vi "Boiler.vi"() -> ()   [LabVIEW 2013]
doc: "This VI is a simulaton of boiler startup controller which allow the user to Start up and Shutdown a boiler.\n\nThe controls on the front panal is to- \n-Start up \n-Simulate the cindition in system and\n-Shut down .\nThe indicators on the front panal is to-\n-Display the status and current step in the startup\n-Display the Shut down process\n-Shoe the elapsed time\n\nThis controller also log event the event as thry occur.\n\nSequence of operation:\n-Start(Application Run): This will start the application and initialize all the controls and indicator.\n-Reset Lockout: This will ready the boiler (It will happen only when Run interlock is in off position).\n-Pre-Purge: On pressing Start sequence this will run for 10 sec.\n-Pilot: On pressing pilot and it will start when Flame senseor value is more than 30%.\n-Shutdown: On pressing it the boiler will go in shut down and it can be done in four ways-\n>shutdoen is clicked\n>Fuel controller value is less than 10% or greater than 75%\n>Run itnterlock switch open.\n>Forced draft switch Off."
uses:
  Controls/Boiler Controls.ctl
  Controls/Boiler Simulation Controls.ctl
  Controls/Boiler Status Indicators.ctl
  Controls/Boiler Application Controls.ctl
  Controls/Boiler States.ctl
panel:
  in  "Stop":T1
  out "Boiler Status Indicators":T2 {"Time Count" format="%.2g"}
  in  "Boiler Simulation Controls":T3 {"Flame Sensor Value (%)" min=0.0 max=100.0 scale=0.0..100.0}
  in  "Boiler Controls":T4 {"Fuel Valve Position" min=0.0 max=100.0 scale=0.0..100.0 scale format="%.2f"}
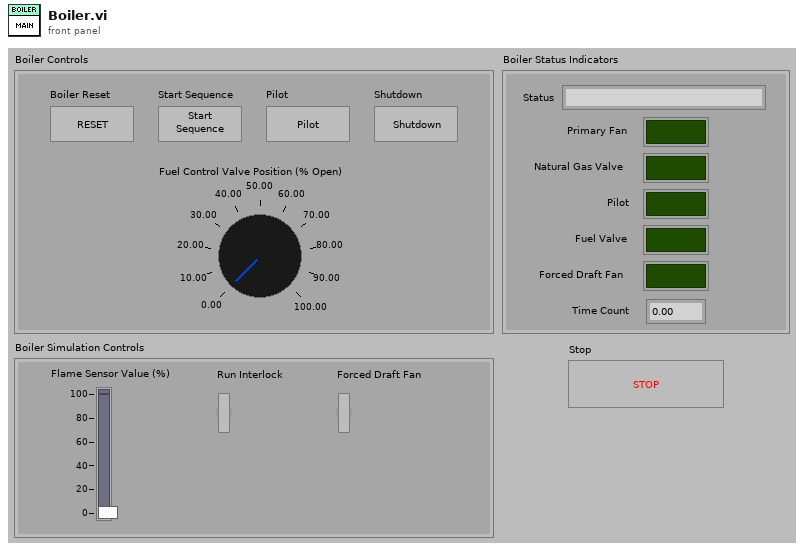
[diagram p1: front panel]
types:
  T1 = typedef "Boiler Application Controls.ctl" = bool
  T2 = typedef "Boiler Status Indicators.ctl" = cluster{"Status":string, "Primary Fan":bool, "Natural Gas Valve":bool, "Pilot":bool, "Fuel Valve":bool, "Forced Draft Fan":bool, "Time Count":dbl}
  T3 = typedef "Boiler Simulation Controls.ctl" = cluster{"Flame Sensor Value (%)":dbl, "Run Interlock":bool, "Forced Draft Fan":bool}
  T4 = typedef "Boiler Controls.ctl" = cluster{"Boiler Reset":bool, "Start Sequence":bool, "Pilot":bool, "Shutdown":bool, "Fuel Valve Position":dbl}
  T5 = typedef "Boiler States.ctl" = enum16{"Initialize", "Reset Lockout", "Pre-Purge", "Pre-Purge(Cont.)", "Ignition", "Prove the pilot", "Start and Run", "Run(Cont.) ", "Shutdown and purge", "Stop"}
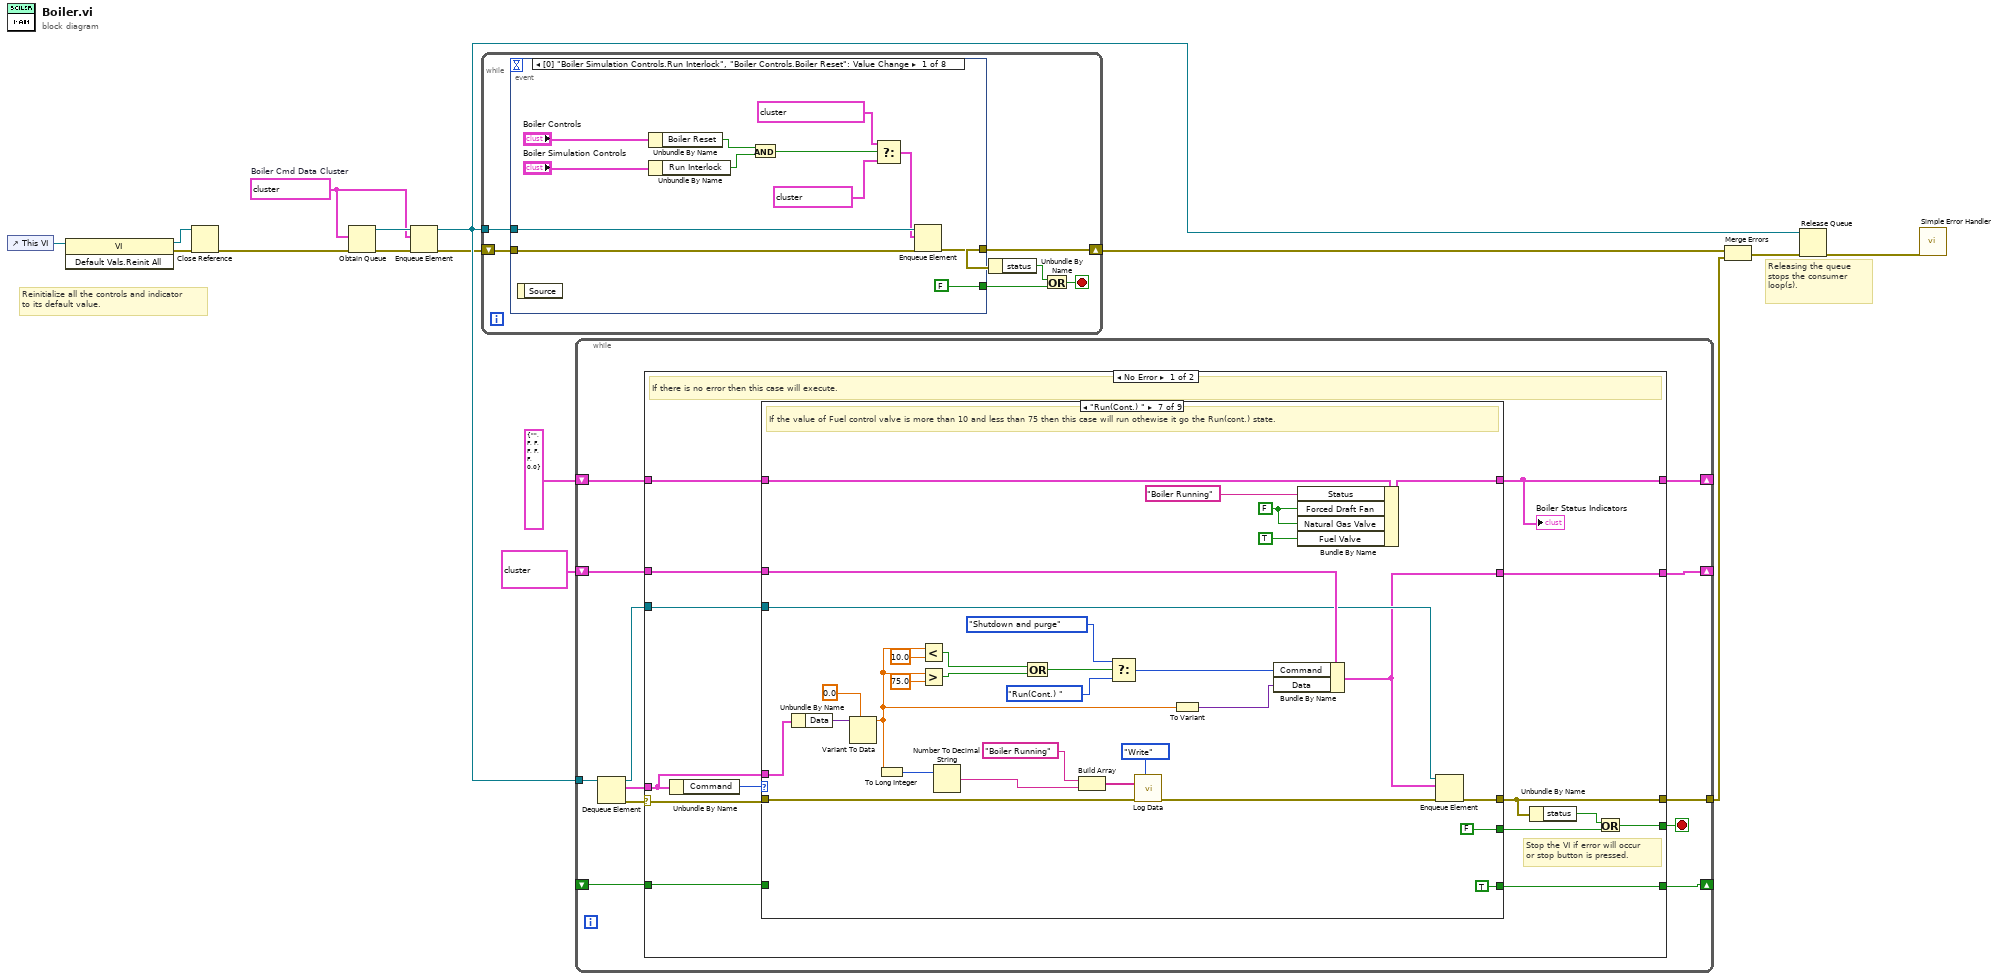
[diagram p0: block diagram]
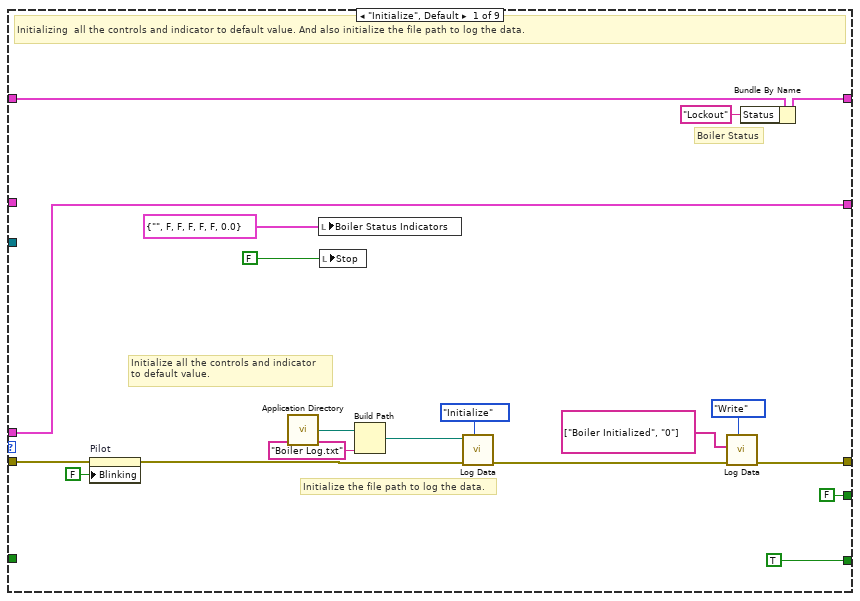
[diagram p2: hidden frame]
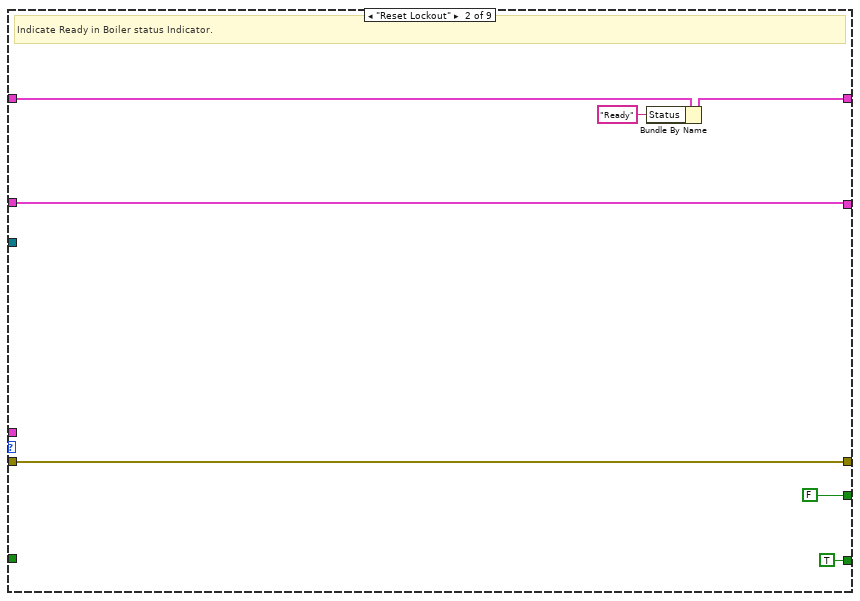
[diagram p3: hidden frame]
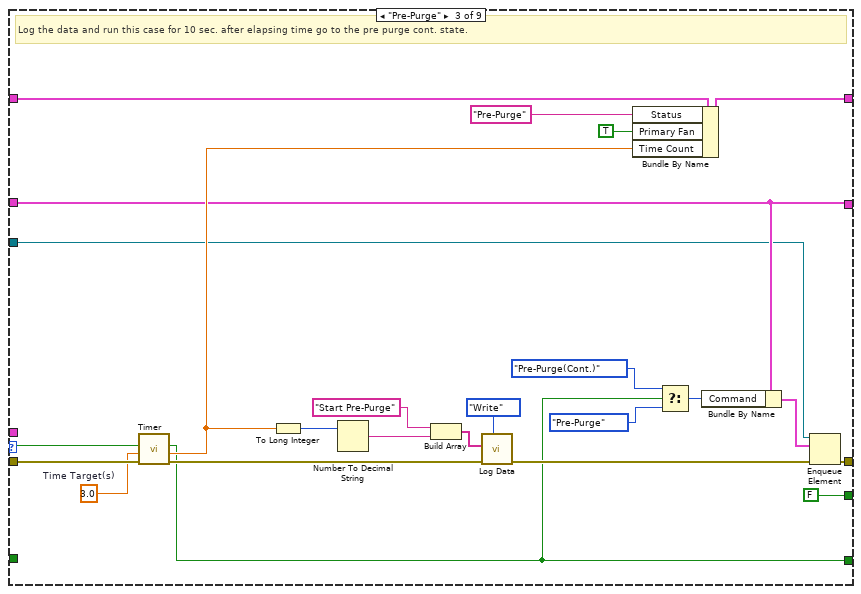
[diagram p4: hidden frame]
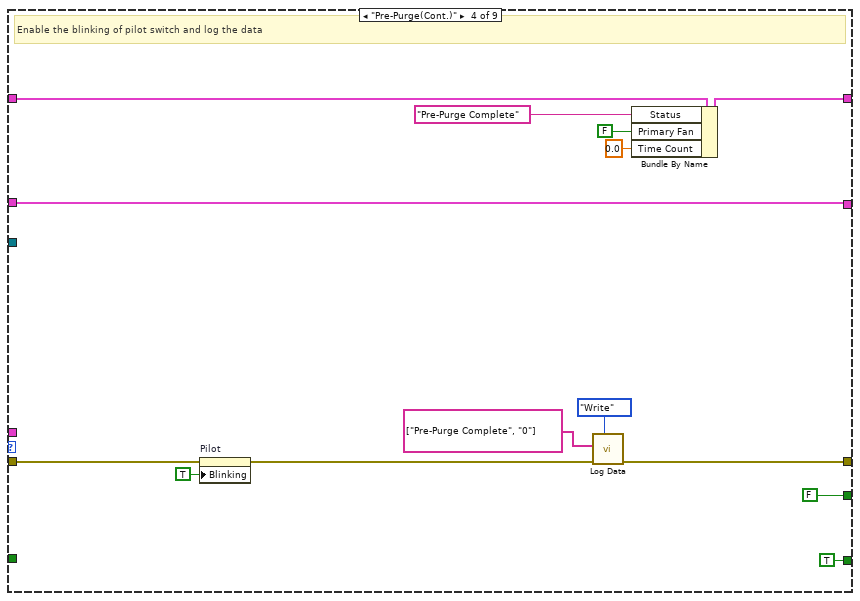
[diagram p5: hidden frame]
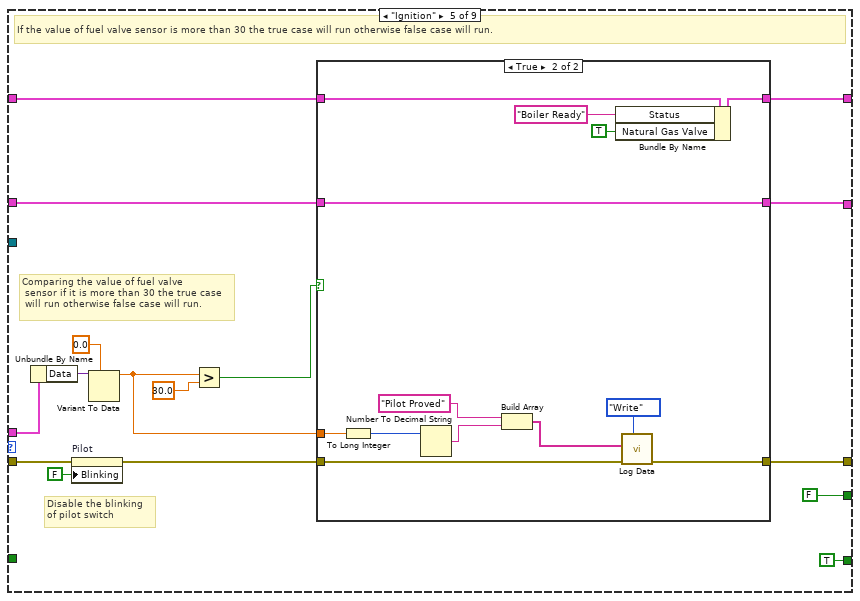
[diagram p6: hidden frame]
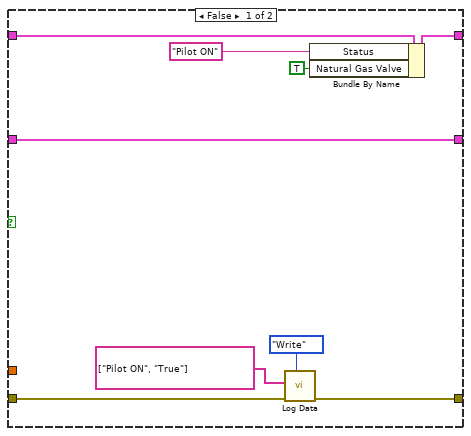
[diagram p7: hidden frame]
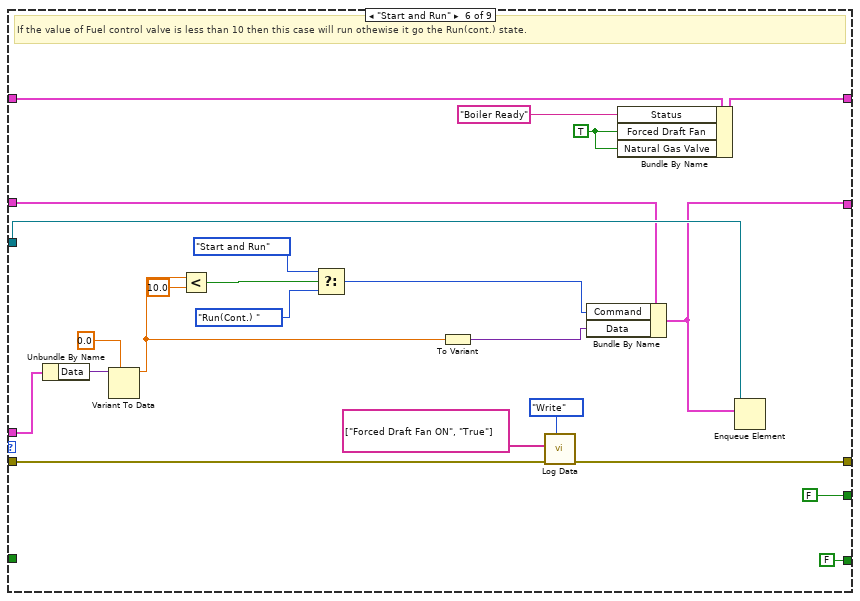
[diagram p8: hidden frame]
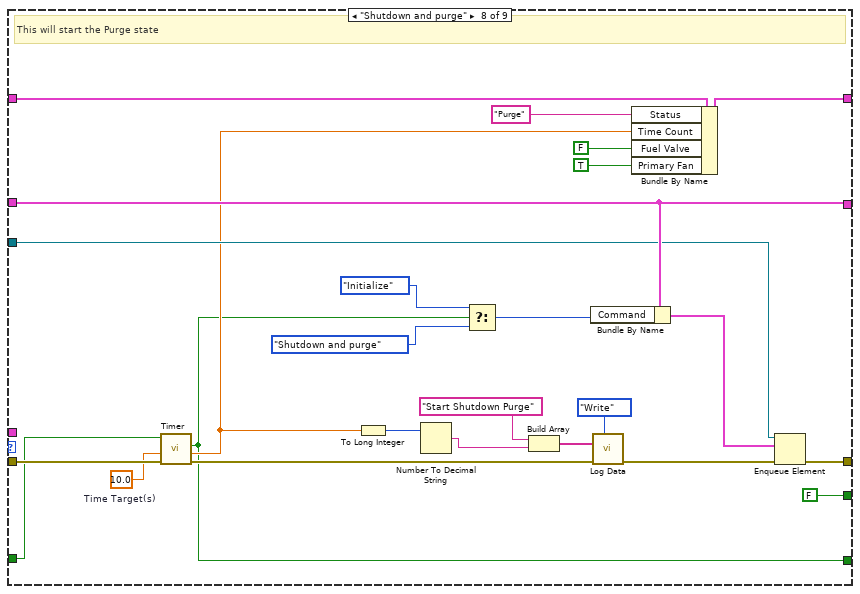
[diagram p9: hidden frame]
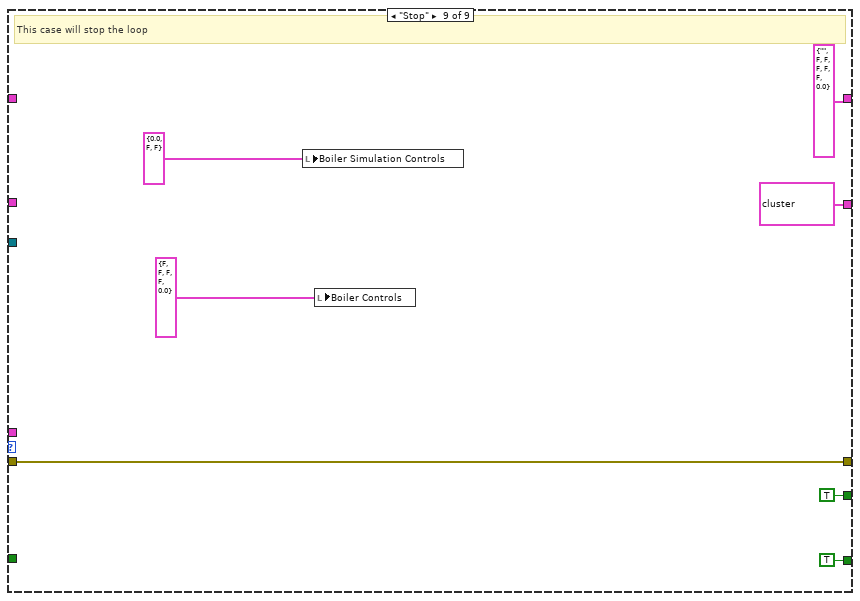
[diagram p10: hidden frame]
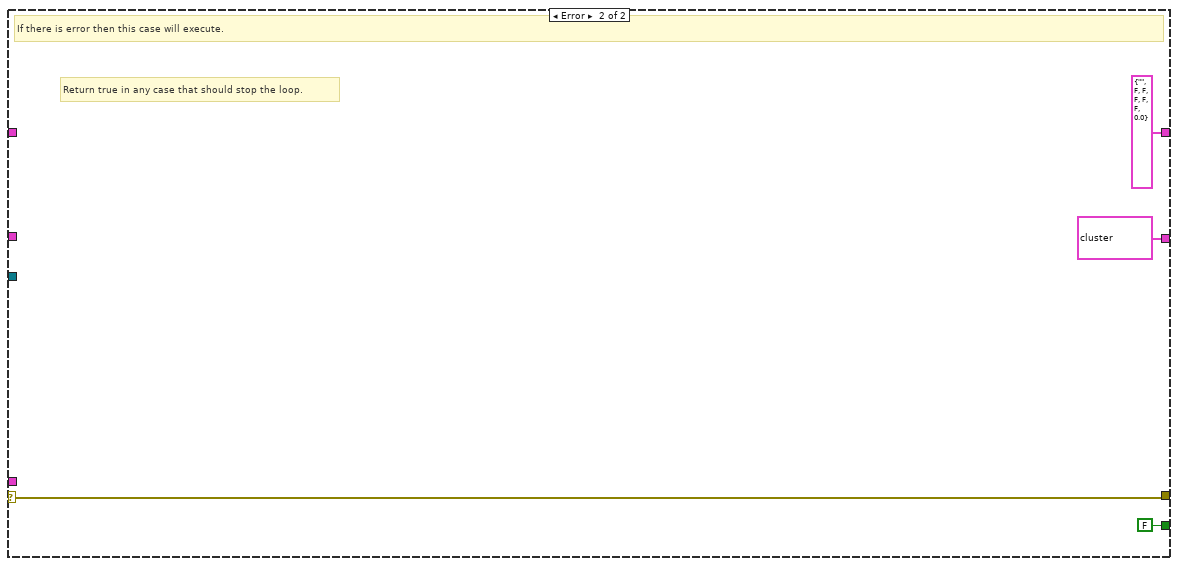
[diagram p11: hidden frame]
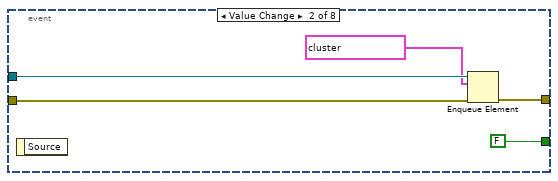
[diagram p12: hidden frame]
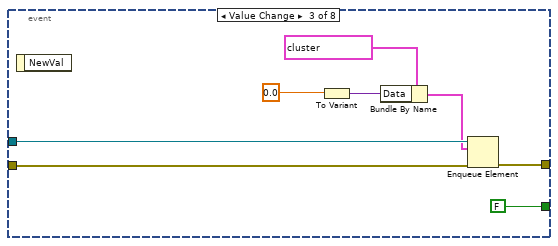
[diagram p13: hidden frame]
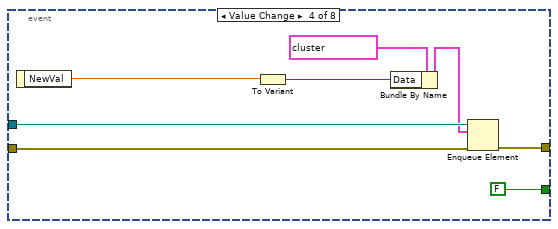
[diagram p14: hidden frame]
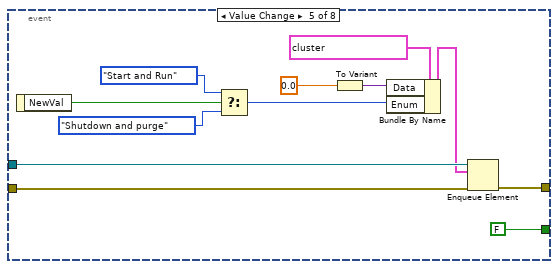
[diagram p15: hidden frame]
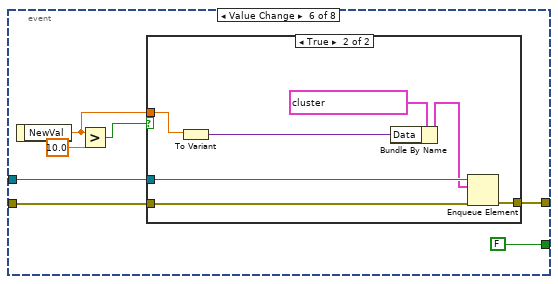
[diagram p16: hidden frame]
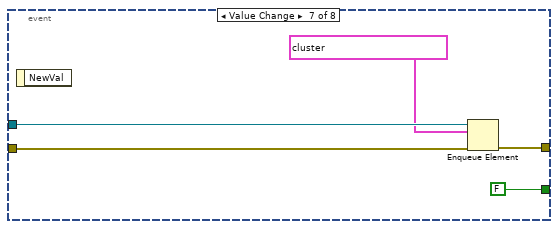
[diagram p18: hidden frame]
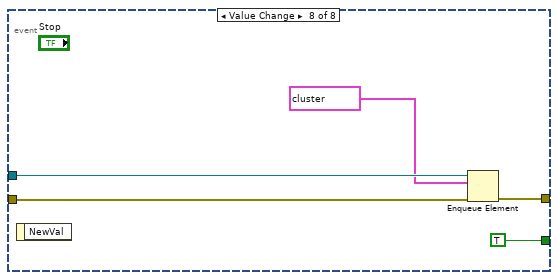
[diagram p19: hidden frame]
diagram:
  w7 = cluster{"Data":variant, "Command":T5} {"Data"=variant, "Command"=enum."Initialize"}  # Boiler Cmd Data Cluster
  # "Reinitialize all the controls and indicator\nto its default value."
  # "Releasing the queue stops the consumer loop(s)."
  n1 = control-ref of="This VI"() -> (w11:refnum<vi>)
  n2 = invoke class="VI" method="Default Vals.Reinit All"(reference=w11) -> (reference out=w9:refnum<vi>, error out=w10:errorcluster)  [unwired: 2 in, 1 out]
  n3 = Close Reference(reference=w9, error in (no error)=w10) -> (error out=w8:errorcluster)
  n4 = Obtain Queue(element data type=w7, error in (no error)=w8) -> (queue out=w15:refnum<queue>, error out=w13:errorcluster)  [unwired: 3 in, 1 out]
  n5 = Enqueue Element(queue=w15, element=w7, error in (no error)=w13) -> (queue out=w14:refnum<queue>, error out=w12:errorcluster)  [unwired: 1 in, 1 out]
  n6 = while {
    shift-right: [w18] -> w6
    shift-left: w12 -> [w20]
    tunnel: w14 -> [w21]
    stop <- w19 stop-if-true
    n7 = event shown="[0] \"Boiler Simulation Controls.Run Interlock\", \"Boiler Controls.Boiler Reset\": Value Change" {
      selector: _ -> [_ _ _ _ _ _ _ _]
      dyn-events: _ -> [_ _ _ _ _ _ _ _]
      timeout: _ -> [_ _ _ _ _ _ _ _]
      tunnel: w21 -> [w31 w36 w44 w52 w64 w71 w84 w89]
      tunnel: w20 -> [w33 w38 w46 w54 w66 w73 w86 w91]
      tunnel: [w32 w37 w45 w53 w65 w72 w85 w90] -> w18
      tunnel: [FALSE FALSE FALSE FALSE FALSE FALSE FALSE TRUE] -> w16
      event Value Change {
        n8 = event-data() -> ()  [unwired: 1 in, 1 out]
        n9 = Unbundle By Name("Boiler Controls") -> ("Boiler Reset"=w28:bool)
        n10 = Unbundle By Name("Boiler Simulation Controls") -> ("Run Interlock"=w29:bool)
        n11 = And(x=w28, y=w29) -> (x .and. y?=w27:bool)
        n12 = Select(t=cluster{"Data":variant, "Enum":T5} {"Data"=variant, "Enum"=enum."Reset Lockout"} ("Boiler Cmd Data Cluster"), s=w27, f=cluster{"Data":variant, "Enum":T5} {"Data"=variant, "Enum"=enum."Initialize"} ("Boiler Cmd Data Cluster")) -> (s? t:f=w24:cluster{"Data":variant, "Enum":T5})
        n13 = Enqueue Element(queue=w31, element=w24, error in (no error)=w33) -> (error out=w32:errorcluster)  [unwired: 1 in, 2 out]
      }
      event Value Change {
        n14 = event-data() -> ()  [unwired: 1 in, 1 out]
        n15 = Enqueue Element(queue=w36, element=cluster{"Data":variant, "Enum":T5} {"Data"=variant, "Enum"=enum."Pre-Purge"} ("Boiler Cmd Data Cluster"), error in (no error)=w38) -> (error out=w37:errorcluster)  [unwired: 1 in, 2 out]
      }
      event Value Change {
        n16 = event-data() -> ()  [unwired: 1 in, 1 out]
        n17 = To Variant(anything=0.0) -> (Variant=w39:variant)
        n18 = Bundle By Name(cluster=cluster{"Data":variant, "Enum":T5} {"Data"=variant, "Enum"=enum."Ignition"} ("Boiler Cmd Data Cluster"), "Data"=w39) -> (w41:cluster{"Data":variant, "Enum":T5})
        n19 = Enqueue Element(queue=w44, element=w41, error in (no error)=w46) -> (error out=w45:errorcluster)  [unwired: 1 in, 2 out]
      }
      event Value Change {
        n20 = event-data() -> ("NewVal"=w48:dbl)  [unwired: 1 in]
        n21 = To Variant(anything=w48) -> (Variant=w47:variant)
        n22 = Bundle By Name(cluster=cluster{"Data":variant, "Enum":T5} {"Data"=variant, "Enum"=enum."Ignition"} ("Boiler Cmd Data Cluster"), "Data"=w47) -> (w49:cluster{"Data":variant, "Enum":T5})
        n23 = Enqueue Element(queue=w52, element=w49, error in (no error)=w54) -> (error out=w53:errorcluster)  [unwired: 1 in, 2 out]
      }
      event Value Change {
        n24 = event-data() -> ("NewVal"=w55:bool)  [unwired: 1 in]
        n25 = Select(t=Boiler_States."Start and Run" ("Enum"), s=w55, f=Boiler_States."Shutdown and purge" ("Enum")) -> (s? t:f=w56:T5)
        n26 = To Variant(anything=0.0) -> (Variant=w60:variant)
        n27 = Bundle By Name(cluster=cluster{"Data":variant, "Enum":T5} {"Data"=variant, "Enum"=enum."Start and Run"} ("Boiler Cmd Data Cluster"), "Data"=w60, "Enum"=w56) -> (w61:cluster{"Data":variant, "Enum":T5})
        n28 = Enqueue Element(queue=w64, element=w61, error in (no error)=w66) -> (error out=w65:errorcluster)  [unwired: 1 in, 2 out]
      }
      event Value Change {
        n29 = event-data() -> ("NewVal"=w67:dbl)  [unwired: 1 in]
        n30 = Greater?(x=w67, y=10.0) -> (0:w68:bool)
        n31 = case shown="True" w68 {
          tunnel: w73 -> [w74 w81]
          tunnel: [w74 w80] -> w72
          tunnel: w71 -> [_ w79]
          tunnel: w67 -> [_ w75]
          frame False {
          }
          frame True {
            n32 = To Variant(anything=w75) -> (Variant=w76:variant)
            n33 = Bundle By Name(cluster=cluster{"Data":variant, "Enum":T5} {"Data"=variant, "Enum"=enum."Start and Run"} ("Boiler Cmd Data Cluster"), "Data"=w76) -> (w77:cluster{"Data":variant, "Enum":T5})
            n34 = Enqueue Element(queue=w79, element=w77, error in (no error)=w81) -> (error out=w80:errorcluster)  [unwired: 1 in, 2 out]
          }
        }
      }
      event Value Change {
        n35 = event-data() -> ()  [unwired: 1 in, 1 out]
        n36 = Enqueue Element(queue=w84, element=cluster{"Data":variant, "Enum":T5} {"Data"=variant, "Enum"=enum."Shutdown and purge"} ("Boiler Cmd Data Cluster"), error in (no error)=w86) -> (error out=w85:errorcluster)  [unwired: 1 in, 2 out]
      }
      event Value Change {
        n37 = event-data() -> ()  [unwired: 1 in, 1 out]
        n38 = Enqueue Element(queue=w89, element=cluster{"Data":variant, "Enum":T5} {"Data"=variant, "Enum"=enum."Stop"} ("Boiler Cmd Data Cluster"), error in (no error)=w91) -> (error out=w90:errorcluster)  [unwired: 1 in, 2 out]
      }
    }
    n39 = Unbundle By Name(w18) -> ("status"=w17:bool)
    n40 = Or(x=w17, y=w16) -> (x .or. y?=w19:bool)
  }
  n41 = while {
    tunnel: w14 -> [w103]
    tunnel: [w100] -> w4
    shift-right: [w98] -> _
    shift-left: T2 {"Status"="", "Primary Fan"=FALSE, "Natural Gas Valve"=FALSE, "Pilot"=FALSE, "Fuel Valve"=FALSE, "Forced Draft Fan"=FALSE, "Time Count"=0.0} ("Boiler Status Indicators") -> [w97]
    shift-right: [w96] -> _
    shift-left: _ -> [w95]
    shift-right: [w94] -> _
    shift-left: cluster{"Data":variant, "Command":T5} {"Data"=variant, "Command"=enum."Initialize"} ("Boiler Cmd Data Cluster") -> [w93]
    stop <- w99 stop-if-true
    n42 = Dequeue Element(queue=w103) -> (queue out=w92:refnum<queue>, element=w101:cluster{"Data":variant, "Command":T5}, error out=w102:errorcluster)  [unwired: 2 in, 1 out]
    n43 = case shown="No Error" w102 {
      selector: w102 -> [w117 w309]
      tunnel: w101 -> [w106 _]
      tunnel: [w116 w309] -> w100
      tunnel: [w113 FALSE] -> w99
      tunnel: [w110 T2 {"Status"="", "Primary Fan"=FALSE, "Natural Gas Valve"=FALSE, "Pilot"=FALSE, "Fuel Valve"=FALSE, "Forced Draft Fan"=FALSE, "Time Count"=0.0} ("Boiler Status Indicators")] -> w98
      tunnel: w97 -> [w111 _]
      tunnel: [w109 _] -> w96
      tunnel: w95 -> [w108 _]
      tunnel: [w107 cluster{"Data":variant, "Command":T5} {"Data"=variant, "Command"=enum."Initialize"} ("Boiler Cmd Data Cluster")] -> w94
      tunnel: w93 -> [w105 _]
      tunnel: w92 -> [w104 _]
      frame No Error {
        # "Stop the VI if error will occur \nor stop button is pressed."
        # "If there is no error then this case will execute."
        n44 = Unbundle By Name(w106) -> ("Command"=w112:T5)
        n45 = case shown="\"Run(Cont.) \"" w112 {
          tunnel: [w125 w143 w151 w169 w187 w231 w261 w292 w303] -> w116
          tunnel: w117 -> [w121 w143 w162 w172 w194 w234 w267 w282 w303]
          tunnel: [FALSE FALSE FALSE FALSE FALSE FALSE FALSE FALSE TRUE] -> w114
          tunnel: [w135 w140 w165 w179 w195 w240 w271 w296 T2 {"Status"="", "Primary Fan"=FALSE, "Natural Gas Valve"=FALSE, "Pilot"=FALSE, "Fuel Valve"=FALSE, "Forced Draft Fan"=FALSE, "Time Count"=0.0} ("Boiler Status Indicators")] -> w110
          tunnel: w111 -> [w136 w141 w166 w180 w196 w241 w272 w297 _]
          tunnel: [TRUE TRUE ("Boolean") w144 TRUE ("Boolean") TRUE ("Boolean") FALSE ("Boolean") TRUE ("Boolean") w274 TRUE ("Boolean")] -> w109
          tunnel: w108 -> [_ _ w161 _ _ _ _ w280 _]
          tunnel: [w122 w137 w150 w175 w183 w220 w248 w291 cluster{"Data":variant, "Command":T5} {"Data"=variant, "Command"=enum."Initialize"} ("Boiler Cmd Data Cluster")] -> w107
          tunnel: w106 -> [w122 _ _ _ w191 w239 w266 _ _]
          tunnel: w105 -> [_ w137 w150 w175 w184 w229 w260 w291 _]
          tunnel: w104 -> [_ _ w148 _ _ w230 w256 w289 _]
          frame "Initialize", Default {
            # "Boiler Status"
            # "Initialize the file path to log the data."
            # "Initialize all the controls and indicator \nto default value."
            # "Initializing  all the controls and indicator to default value. And also initialize the file path to log the data."
            n46 = property on="Pilot" class="Bool (strict)"(error in=w121, "Blinking"=FALSE) -> (error out=w120:errorcluster)  [unwired: 1 in, 1 out]
            n47 = call <vilib>:"Application Directory.vi"() -> ("Application Directory"=w130:path)
            n48 = local write "Boiler Status Indicators"(T2 {"Status"="", "Primary Fan"=FALSE, "Natural Gas Valve"=FALSE, "Pilot"=FALSE, "Fuel Valve"=FALSE, "Forced Draft Fan"=FALSE, "Time Count"=0.0} ("Boiler Status Indicators")) -> ()
            n49 = local write "Stop"(T1 FALSE ("Stop")) -> ()
            n50 = Build Path(base path=w130, name or relative path="Boiler Log.txt") -> (appended path=w129:path)
            n51 = call "Log Data.vi"("Command"=enum16{"Initialize", "Write", "Stop"}."Initialize", "error in (no error)"=w120, "file path"=w129) -> ("error out"=w126:errorcluster)  [unwired: 8 in]
            n52 = call "Log Data.vi"("Command"=enum16{"Initialize", "Write", "Stop"}."Write", "error in (no error)"=w126, "Event Data"=string[] ["Boiler Initialized", "0"]) -> ("error out"=w125:errorcluster)  [unwired: 8 in]
            n53 = Bundle By Name(cluster=w136, "Status"="Lockout") -> (w135:T2)
          }
          frame "Reset Lockout" {
            # "Indicate Ready in Boiler status Indicator."
            n54 = Bundle By Name(cluster=w141, "Status"="Ready") -> (w140:T2)
          }
          frame "Pre-Purge" {
            w160 = 3.0  # Time Target(s)
            # "Log the data and run this case for 10 sec. after elapsing time go to the pre purge cont. state."
            n55 = call "Timer.vi"("error in (no error)"=w162, "Time Target(s)"=w160, "Reset"=w161) -> ("error out"=w159:errorcluster, "Elapsed Time"=w157:dbl, "Boolean"=w144:bool)  [unwired: 6 in]
            n56 = To Long Integer(number=w157) -> (32bit integer=w156:i32)
            n57 = Number To Decimal String(number=w156) -> (decimal integer string=w154:string)  [unwired: 1 in]
            n58 = Build Array("Start Pre-Purge", w154) -> (w153:string[])
            n59 = call "Log Data.vi"("Command"=enum16{"Initialize", "Write", "Stop"}."Write", "error in (no error)"=w159, "Event Data"=w153) -> ("error out"=w152:errorcluster)  [unwired: 8 in]
            n60 = Bundle By Name(cluster=w166, "Status"="Pre-Purge", "Primary Fan"=TRUE, "Time Count"=w157) -> (w165:T2)
            n61 = Select(t=Boiler_States."Pre-Purge(Cont.)" ("Command"), s=w144, f=Boiler_States."Pre-Purge" ("Command")) -> (s? t:f=w147:T5)
            n62 = Bundle By Name(cluster=w150, "Command"=w147) -> (w149:cluster{"Data":variant, "Command":T5})
            n63 = Enqueue Element(queue=w148, element=w149, error in (no error)=w152) -> (error out=w151:errorcluster)  [unwired: 1 in, 2 out]
          }
          frame "Pre-Purge(Cont.)" {
            # "Enable the blinking of pilot switch and log the data"
            n64 = property on="Pilot" class="Bool (strict)"(error in=w172, "Blinking"=TRUE) -> (error out=w171:errorcluster)  [unwired: 1 in, 1 out]
            n65 = call "Log Data.vi"("Command"=enum16{"Initialize", "Write", "Stop"}."Write", "error in (no error)"=w171, "Event Data"=string[] ["Pre-Purge Complete", "0"]) -> ("error out"=w169:errorcluster)  [unwired: 8 in]
            n66 = Bundle By Name(cluster=w180, "Status"="Pre-Purge Complete", "Primary Fan"=FALSE, "Time Count"=0.0) -> (w179:T2)
          }
          frame "Ignition" {
            # "Disable the blinking \nof pilot switch"
            # "Comparing the value of fuel valve\n sensor if it is more than 30 the true case\n will run otherwise false case will run."
            # "If the value of fuel valve sensor is more than 30 the true case will run otherwise false case will run."
            n67 = Unbundle By Name(w191) -> ("Data"=w190:variant)
            n68 = property on="Pilot" class="Bool (strict)"(error in=w194, "Blinking"=FALSE) -> (error out=w193:errorcluster)  [unwired: 1 in, 1 out]
            n69 = Variant To Data(type=0.0 ("NewVal"), Variant=w190) -> (data=w185:dbl)  [unwired: 1 in, 1 out]
            n70 = Greater?(x=w185, y=30.0) -> (0:w186:bool)
            n71 = case shown="True" w186 {
              tunnel: w196 -> [w206 w219]
              tunnel: [w205 w218] -> w195
              tunnel: w193 -> [w200 w215]
              tunnel: [w199 w214] -> w187
              tunnel: w185 -> [_ w213]
              tunnel: w184 -> [w198 w208]
              tunnel: [w198 w208] -> w183
              frame False {
                n72 = call "Log Data.vi"("Command"=enum16{"Initialize", "Write", "Stop"}."Write", "error in (no error)"=w200, "Event Data"=string[] ["Pilot ON", "True"]) -> ("error out"=w199:errorcluster)  [unwired: 8 in]
                n73 = Bundle By Name(cluster=w206, "Status"="Pilot ON", "Natural Gas Valve"=TRUE ("Primary Fan")) -> (w205:T2)
              }
              frame True {
                n74 = To Long Integer(number=w213) -> (32bit integer=w212:i32)
                n75 = Number To Decimal String(number=w212) -> (decimal integer string=w210:string)  [unwired: 1 in]
                n76 = Build Array("Pilot Proved", w210) -> (w209:string[])
                n77 = Bundle By Name(cluster=w219, "Status"="Boiler Ready", "Natural Gas Valve"=TRUE) -> (w218:T2)
                n78 = call "Log Data.vi"("Command"=enum16{"Initialize", "Write", "Stop"}."Write", "error in (no error)"=w215, "Event Data"=w209) -> ("error out"=w214:errorcluster)  [unwired: 8 in]
              }
            }
          }
          frame "Start and Run" {
            w232 = TRUE ("Primary Fan")
            # "If the value of Fuel control valve is less than 10 then this case will run othewise it go the Run(cont.) state."
            n79 = Unbundle By Name(w239) -> ("Data"=w238:variant)
            n80 = Variant To Data(type=0.0, Variant=w238) -> (data=w222:dbl)  [unwired: 1 in, 1 out]
            n81 = Less?(x=w222, y=10.0) -> (x < y?=w226:bool)
            n82 = Select(t=Boiler_States."Start and Run" ("Command"), s=w226, f=Boiler_States."Run(Cont.) " ("Command")) -> (s? t:f=w223:T5)
            n83 = To Variant(anything=w222) -> (Variant=w221:variant)
            n84 = call "Log Data.vi"("Command"=enum16{"Initialize", "Write", "Stop"}."Write", "error in (no error)"=w234, "Event Data"=string[] ["Forced Draft Fan ON", "True"]) -> ("error out"=w231:errorcluster)  [unwired: 8 in]
            n85 = Bundle By Name(cluster=w229, "Command"=w223, "Data"=w221) -> (w220:cluster{"Data":variant, "Command":T5})
            n86 = Bundle By Name(cluster=w241, "Status"="Boiler Ready", "Forced Draft Fan"=w232, "Natural Gas Valve"=w232) -> (w240:T2)
            n87 = Enqueue Element(queue=w230, element=w220) -> ()  [unwired: 2 in, 3 out]
          }
          frame "Run(Cont.) " {
            w268 = FALSE ("Primary Fan")
            # "If the value of Fuel control valve is more than 10 and less than 75 then this case will run othewise it go the Run(cont.) state."
            n88 = Unbundle By Name(w266) -> ("Data"=w265:variant)
            n89 = Variant To Data(type=0.0, Variant=w265) -> (data=w247:dbl)  [unwired: 1 in, 1 out]
            n90 = To Long Integer(number=w247) -> (32bit integer=w254:i32)
            n91 = Less?(x=w247, y=10.0) -> (x < y?=w245:bool)
            n92 = Greater?(x=w247, y=75.0) -> (0:w244:bool)
            n93 = Number To Decimal String(number=w254) -> (decimal integer string=w252:string)  [unwired: 1 in]
            n94 = Compound Arithmetic op=OR(w245, w244) -> (w243:bool)
            n95 = Build Array("Boiler Running", w252) -> (w251:string[])
            n96 = Select(t=Boiler_States."Shutdown and purge" ("Command"), s=w243, f=Boiler_States."Run(Cont.) " ("Command")) -> (s? t:f=w259:T5)
            n97 = call "Log Data.vi"("Command"=enum16{"Initialize", "Write", "Stop"}."Write", "error in (no error)"=w267, "Event Data"=w251) -> ("error out"=w262:errorcluster)  [unwired: 8 in]
            n98 = To Variant(anything=w247) -> (Variant=w250:variant)
            n99 = Bundle By Name(cluster=w260, "Command"=w259, "Data"=w250) -> (w248:cluster{"Data":variant, "Command":T5})
            n100 = Bundle By Name(cluster=w272, "Status"="Boiler Running", "Forced Draft Fan"=w268, "Natural Gas Valve"=w268, "Fuel Valve"=TRUE) -> (w271:T2)
            n101 = Enqueue Element(queue=w256, element=w248, error in (no error)=w262) -> (error out=w261:errorcluster)  [unwired: 1 in, 2 out]
          }
          frame "Shutdown and purge" {
            w279 = 10.0  # Time Target(s)
            # "This will start the Purge state"
            n102 = call "Timer.vi"("error in (no error)"=w282, "Time Target(s)"=w279, "Pause"=w280) -> ("error out"=w281:errorcluster, "Elapsed Time"=w278:dbl, "Boolean"=w274:bool)  [unwired: 6 in]
            n103 = To Long Integer(number=w278) -> (32bit integer=w287:i32)
            n104 = Number To Decimal String(number=w287) -> (decimal integer string=w285:string)  [unwired: 1 in]
            n105 = Select(t=Boiler_States."Initialize" ("Command"), s=w274, f=Boiler_States."Shutdown and purge" ("Command")) -> (s? t:f=w275:T5)
            n106 = Build Array("Start Shutdown Purge", w285) -> (w284:string[])
            n107 = Bundle By Name(cluster=w291, "Command"=w275) -> (w290:cluster{"Data":variant, "Command":T5})
            n108 = call "Log Data.vi"("Command"=enum16{"Initialize", "Write", "Stop"}."Write", "error in (no error)"=w281, "Event Data"=w284) -> ("error out"=w293:errorcluster)  [unwired: 8 in]
            n109 = Bundle By Name(cluster=w297, "Status"="Purge", "Time Count"=w278, "Fuel Valve"=FALSE, "Primary Fan"=TRUE) -> (w296:T2)
            n110 = Enqueue Element(queue=w289, element=w290, error in (no error)=w293) -> (error out=w292:errorcluster)  [unwired: 1 in, 2 out]
          }
          frame "Stop" {
            # "This case will stop the loop"
            n111 = local write "Boiler Simulation Controls"(T3 {"Flame Sensor Value (%)"=0.0, "Run Interlock"=FALSE, "Forced Draft Fan"=FALSE} ("Boiler Simulation Controls")) -> ()
            n112 = local write "Boiler Controls"(T4 {"Boiler Reset"=FALSE, "Start Sequence"=FALSE, "Pilot"=FALSE, "Shutdown"=FALSE, "Fuel Valve Position"=0.0} ("Boiler Controls")) -> ()
          }
        }
        "Boiler Status Indicators" <- w110
        n113 = Unbundle By Name(w116) -> ("status"=w115:bool)
        n114 = Or(x=w115, y=w114) -> (x .or. y?=w113:bool)
      }
      frame Error {
        # "Return true in any case that should stop the loop."
        # "If there is error then this case will execute."
      }
    }
  }
  n115 = Merge Errors(w6, w4) -> (w5:errorcluster)
  n116 = Release Queue(queue=w14, error in (no error)=w5) -> (error out=w1:errorcluster)  [unwired: 1 in, 2 out]
  n117 = call <vilib>:"Simple Error Handler.vi"("error in (no error)"=w1) -> ()  [unwired: 4 in, 5 out]
